vi "Read Data as Mono10 to Mono16 Image.vi"(8 "error in (no error)":errorcluster, 11 "Buffer in":refnum<class "Buffer.lvclass">) -> (0 "error out":errorcluster, 2 "Image":u16[][](array[numeric]), 3 "Buffer":refnum<class "Buffer.lvclass">)   [LabVIEW 2020, in "Buffer.lvclass"]
uses:
  Buffer.lvclass
  Buffer.lvclass/Buffer.ctl
  bin/gindustrialcam_32-1.dll
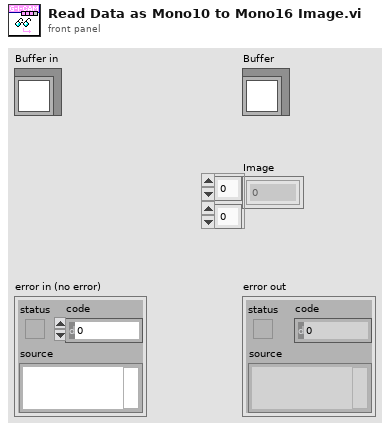
[diagram p1: front panel]
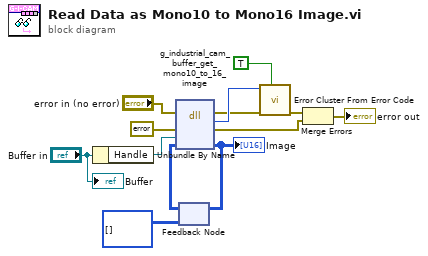
[diagram p0: block diagram]
diagram:
  n1 = Unbundle By Name("Buffer in") -> ("Handle"=w1:refnum<data-value>)
  n2 = feedback #1(u16[][] [] ("Image")) -> (w3:u16[][])
  n3 = dll-call lib="C:/serenial/lib/g-industrial-camera/LabVIEW/g_industrial_cam/bin/gindustrialcam_*-1.*" fn="g_industrial_cam_buffer_get_mono10_to_16_image"(error in="error in (no error)", "err"=errorcluster {"status"=FALSE, "code"=0, "source"=""} ("error constant"), "edvr"=w1, "Image"=w3) -> (error out=w7:errorcluster, "Mg_Error"=w8:i32, "err"=w10:errorcluster, "Image"=w4:u16[][])  [unwired: 3 in, 1 out]
  "Image" <- w4
  n4 = feedback-in #1(w4) -> ()
  n5 = call <vilib>:"Error Cluster From Error Code.vi"("show call chain? (False)"=TRUE, "error in (no error)"=w7, "error code (0)"=w8) -> ("error out"=w9:errorcluster)  [unwired: 6 in]
  n6 = Merge Errors(w9, w10) -> (→"error out":errorcluster)
  "Buffer" <- "Buffer in"
